vi "CreateClass.vi"(0 "ClassWriterGOOP400.lvclass":refnum<class "ClassWriterGOOP400.lvclass">, 1 "ProjectTreePosition(String or Project Item Ref)":variant, 2 "CreateClassData":T1, 5 "error in (no error)":errorcluster, 6 "KeepLvClassRefOpen(False)":bool, 7 "HeaderToApply (take from VIRef or /use 2D-8bit header, Ignored if not wired)":variant) -> (14 "ClassWriterGOOP400.lvclass":refnum<class "ClassWriterGOOP400.lvclass">, 15 "LVClassLibraryRefnum":refnum<vi>, 16 "TemplateVersionUsed":string, 19 "error out":errorcluster)   [LabVIEW 2012, in "ClassWriterGOOP400.lvclass"]
uses:
  <resource>/Framework/Providers/Open_GDS/ClassProviders/Provider_EndevoGOOP400/ClassWriterGOOP400_class/ClassWriterGOOP400.lvclass
  <resource>/Framework/Providers/Open_GDS/ClassProviders/Provider_BaseClassInterface/CreateClassData.ctl
  <resource>/Framework/Providers/Open_GDS/ClassProviders/Provider_EndevoGOOP400/EndevoG4ProviderName.ctl
  <resource>/Framework/Providers/Open_GDS/ClassProviders/Common/LvClass_class/GDSLvCLass_ClassSettingsType.ctl
  <resource>/Framework/Providers/Open_GDS/ClassProviders/Common/LvClass_class/GDSLvClass_PlugIn.ctl
  <resource>/Framework/Providers/Open_GDS/ClassProviders/Common/LvClass_class/GDSLvClass_PlugInTypes.ctl
  <resource>/Framework/Providers/Open_GDS/ClassProviders/Provider_BaseClassInterface/ClassWriter_class/ClassWriter.lvclass
  <resource>/Framework/Providers/Open_GDS/ClassProviders/Provider_LvNativeClass/ClassWriterNative_class/ClassWriterNative.lvclass
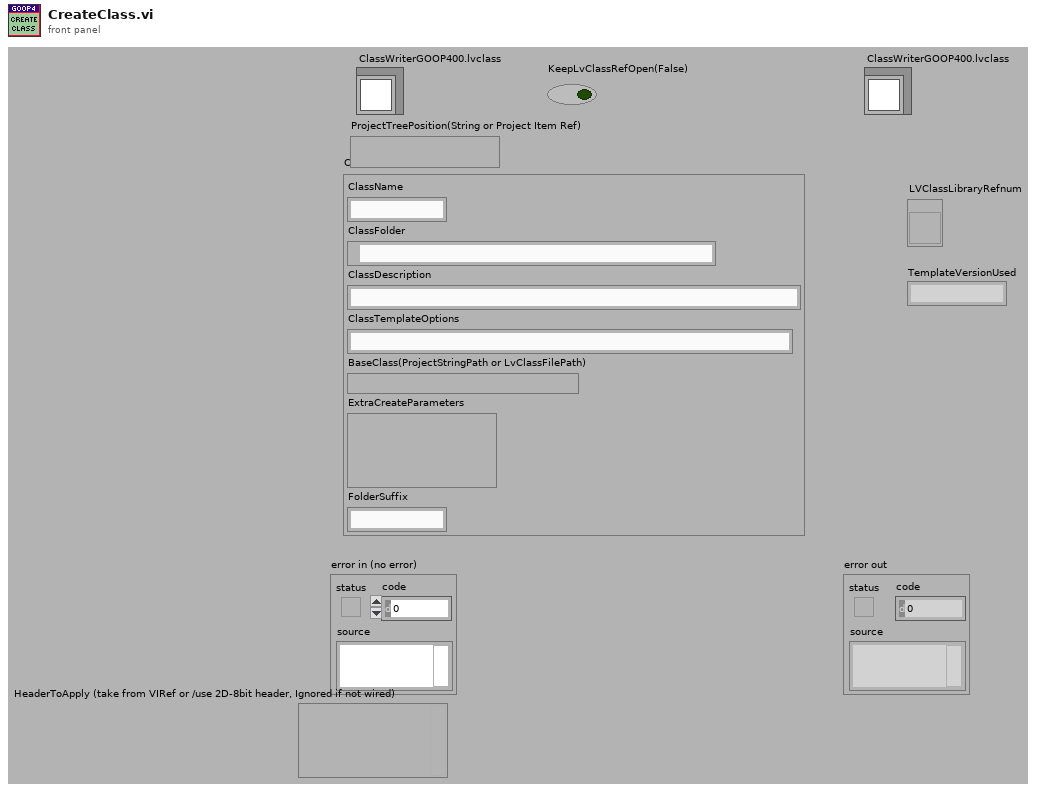
[diagram p1: front panel]
types:
  T1 = typedef "ClassWriter.lvclass/CreateClassData.ctl" = cluster{"ClassName":string, "ClassFolder":path, "ClassDescription":string, "ClassTemplateOptions":string, "BaseClass(ProjectStringPath or LvClassFilePath)":variant, "ExtraCreateParameters":variant, "FolderSuffix":string}
  T2 = cluster{"SubClass":bool, "ClassTemplateFiles":path[], "ClassName":string, "ClassFolder":path, "VIs":refnum<vi>[], "TemplateFolder":path, "ViSubDirs":string[], "TemplateName":string, "BaseClassFolder":path, "RootBaseClassFolder":path, "LvClassPath":path, "ClassRefnum":refnum<vi>, "ProjectRefnum":refnum<vi>, "LvClassFolderPath":path, "BaseClassName":string, "ClassItems":refnum<vi>[], "ViLocked":bool[], "ProjectItemOwner":refnum<vi>, "DeleteFiles":path[], "VIsBefore":refnum<vi>[], "BaseClassPath":path, "BaseConstructorBase":path, "TemplBaseConstructorBase":path, "TemplatePath":path, "TemplateVersion":string, "TemplateParentClass":refnum<vi>, "App":refnum<vi>, "Parent Class":refnum<vi>, "ParentVIs":refnum<vi>[], "TempClass":refnum<vi>}
  T3 = typedef "EndevoG4ProviderName.ctl" = enum16{"EndevoGOOP400"}
  T4 = typedef "GDSLvCLass_ClassSettingsType.ctl" = cluster{"ClassProviderName":string, "ClassTemplateUsed":string, "ClassTemplateVersion":string, "ClassDescription":string, "PlugIns":T5[], "ConnectorPanePattern":string}
  T5 = typedef "GDSLvClass_PlugIn.ctl" = cluster{"Type":T6, "ID":string, "Version":string, "Path":path, "Name":string, "Data":variant}
  T6 = typedef "GDSLvClass_PlugInTypes.ctl" = enum16{"DesignPattern", "MethodTypes"}
  T7 = enum32{"invalid scope", "public", "private", "protected"}
  T8 = enum32{"invalid lock state", "Not Locked", "Locked (No Password)", "Password-protected"}
  T9 = typedef "ClassWriter.lvclass/TemplateSettings.ctl" = cluster{"CommonClassTemplate":bool, "DynamicDispatch":enum8{"False", "True", "Mixed"}, "MustOverride":enum8{"False", "True", "Mixed"}, "MustCallParent":enum8{"False", "True", "Mixed"}, "OnlyNormalMethod":bool, "OnlyPublic":bool}
  T10 = cluster{"Major":u16, "Minor":u16, "Fix":u16, "Build":u16}
  T11 = typedef "Scripting_ConnectorPanePatternType.ctl" = u16
  T12 = typedef "GOOP400_Options.ctl" = cluster{"FlatFolderStructure":bool}
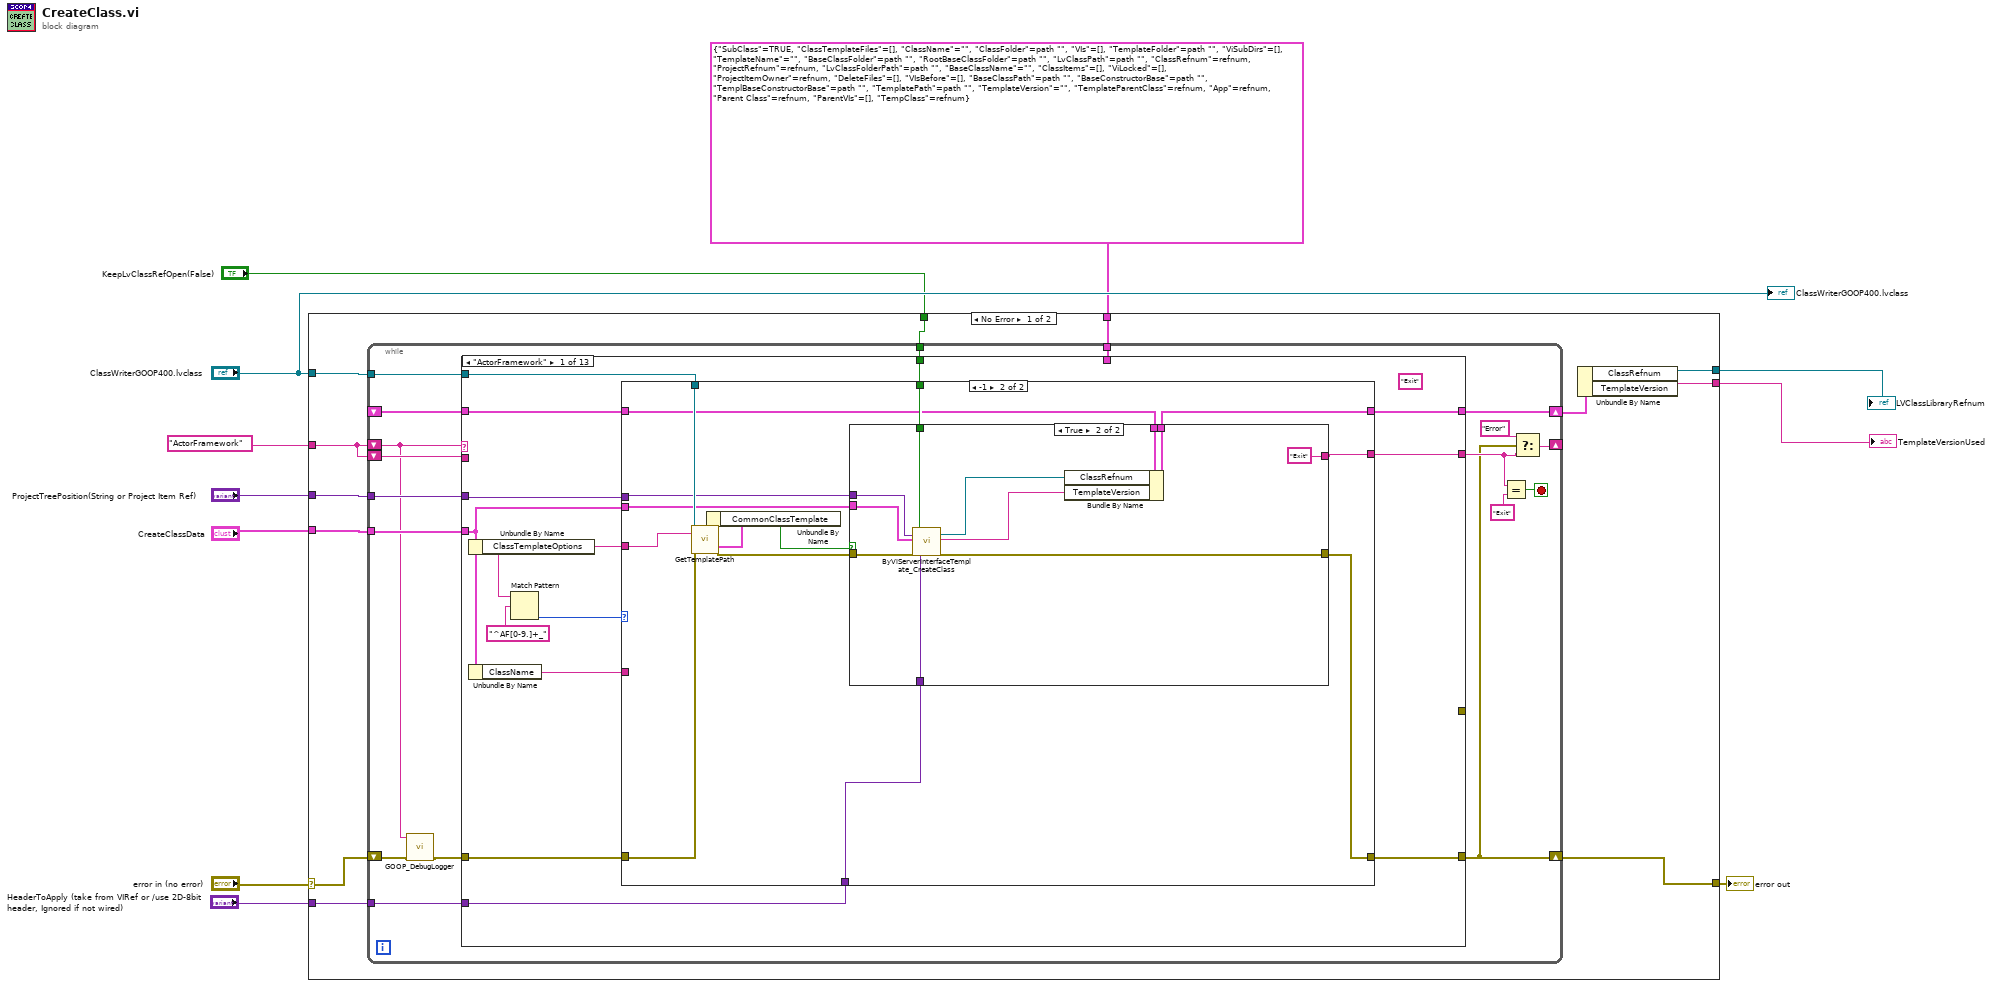
[diagram p0: block diagram]
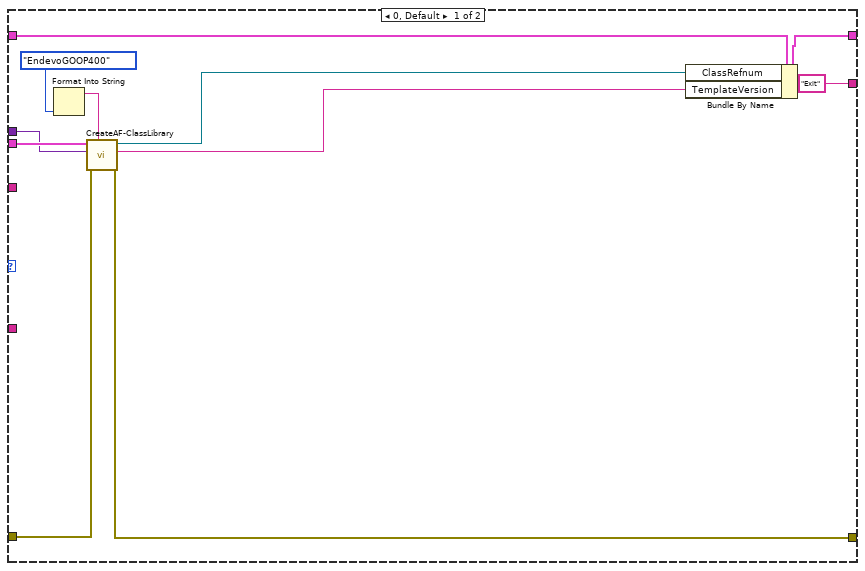
[diagram p2: hidden frame]
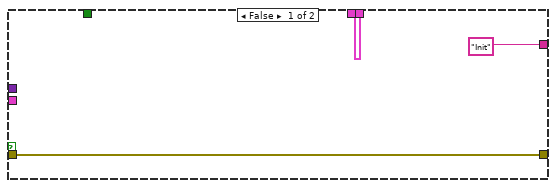
[diagram p3: hidden frame]
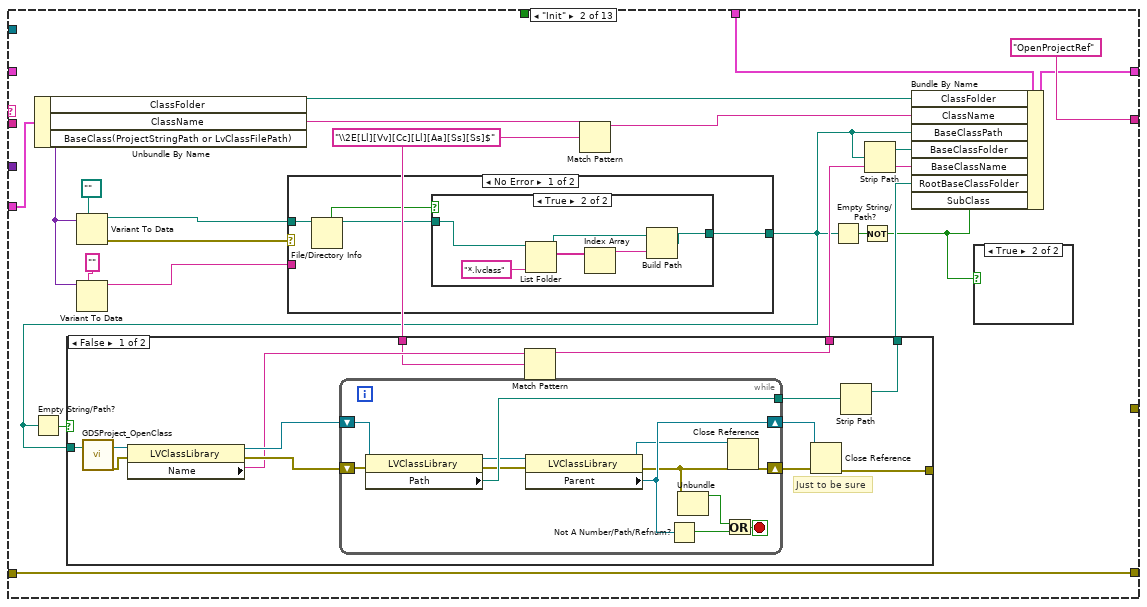
[diagram p4: hidden frame]
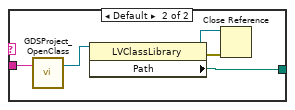
[diagram p9: hidden frame]
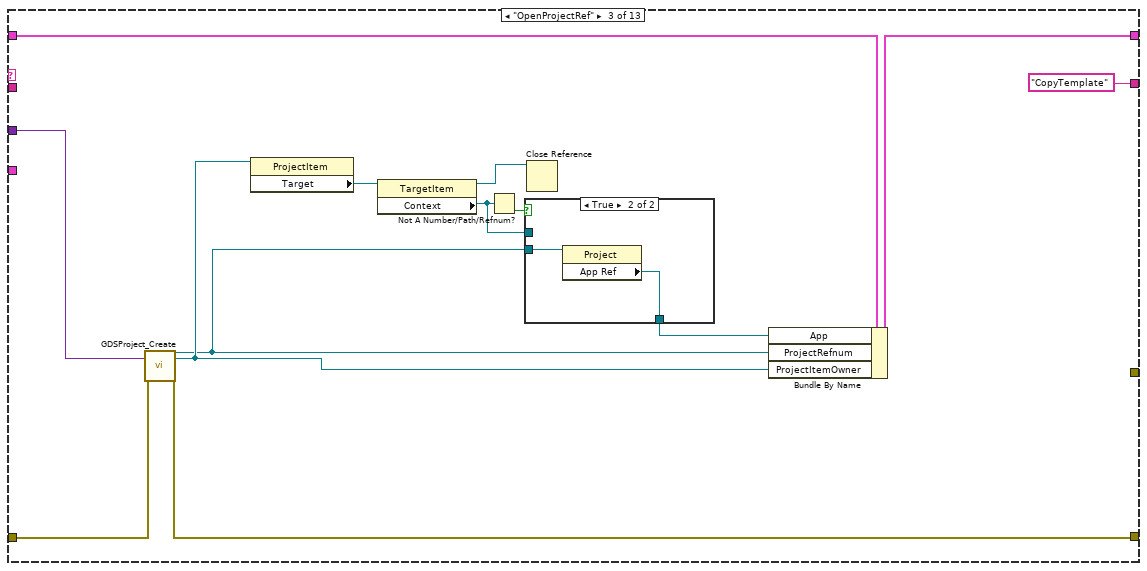
[diagram p10: hidden frame]
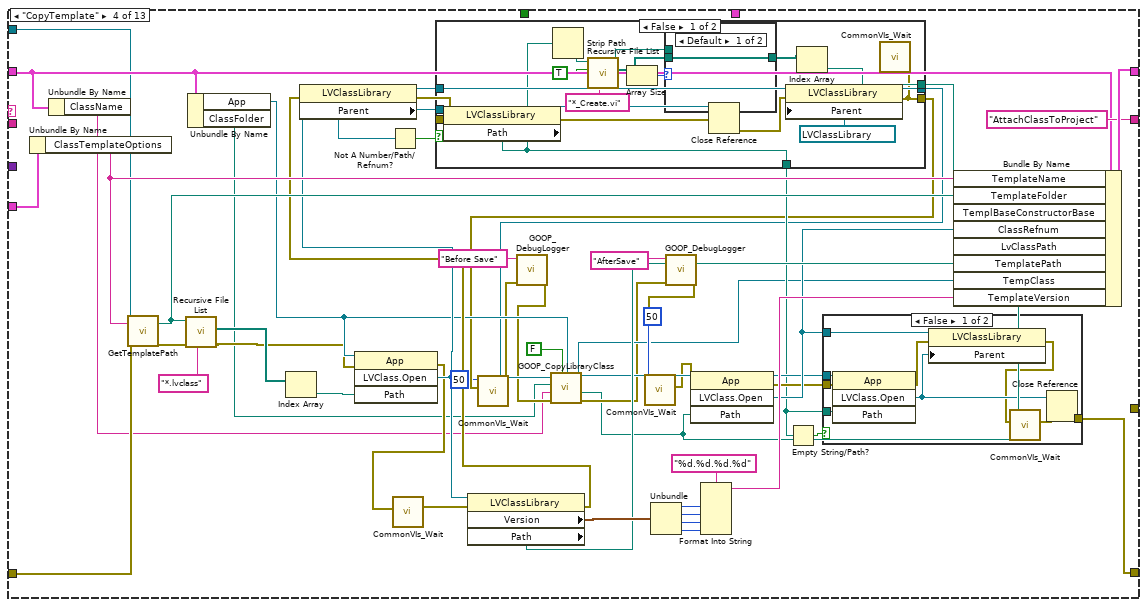
[diagram p12: hidden frame]
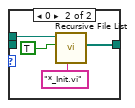
[diagram p14: hidden frame]
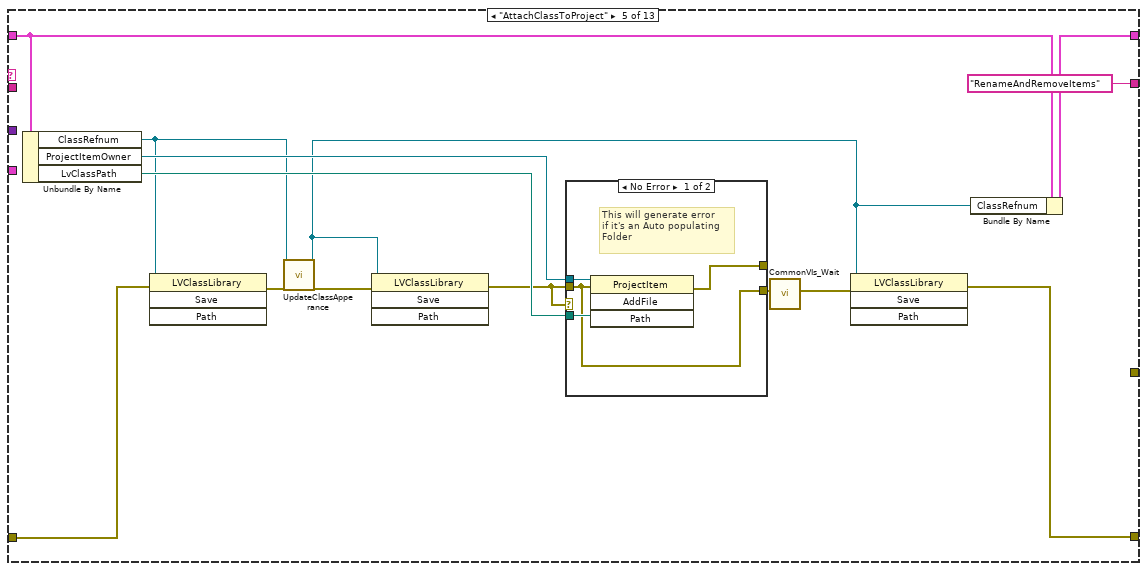
[diagram p16: hidden frame]
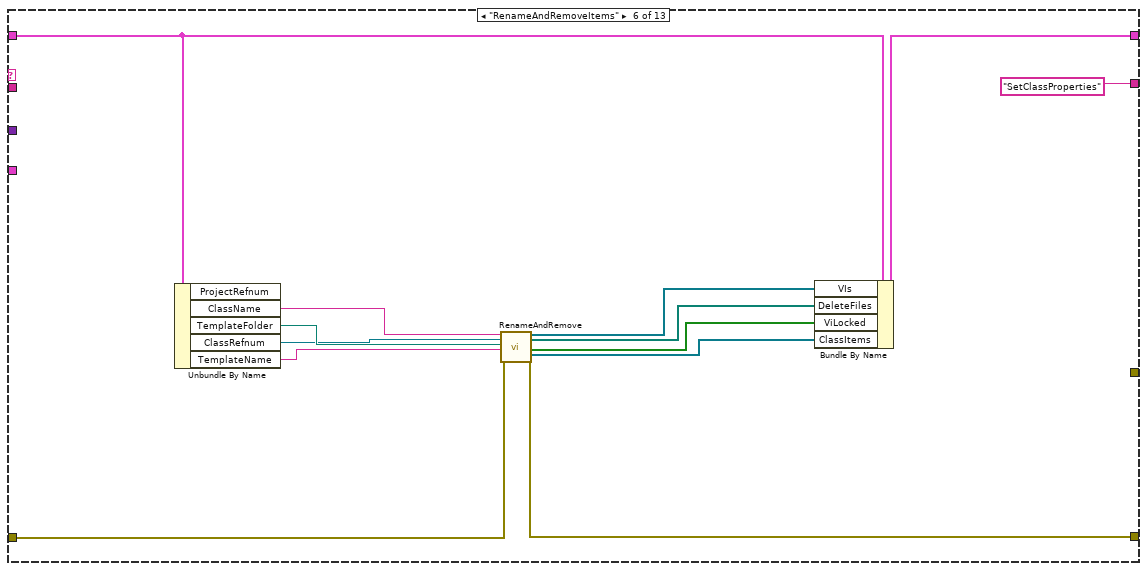
[diagram p18: hidden frame]
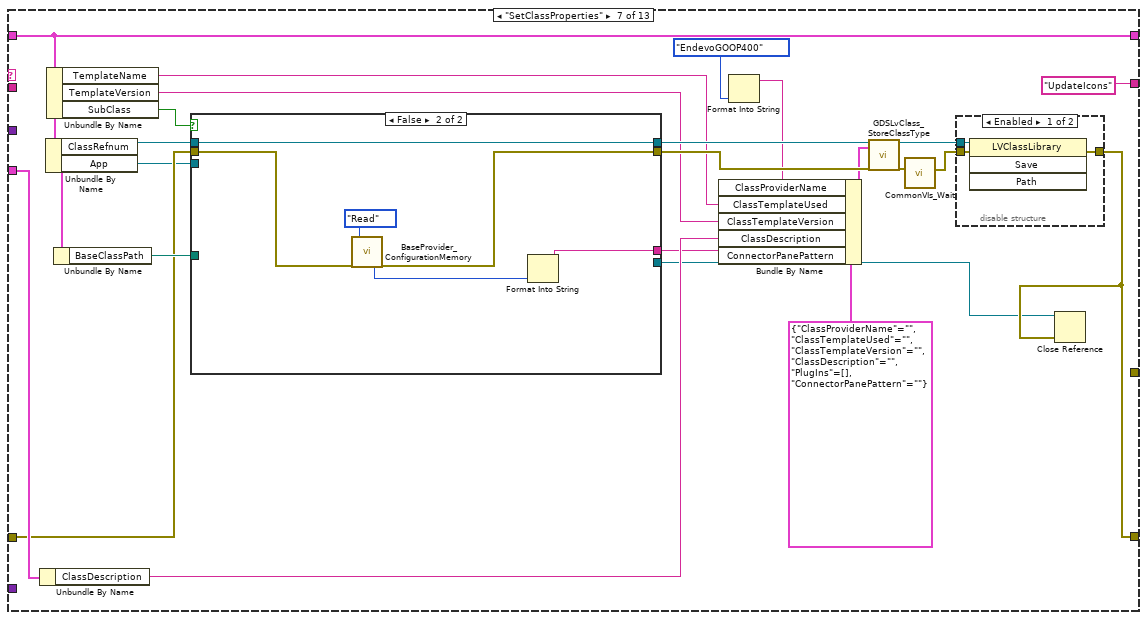
[diagram p19: hidden frame]
diagram:
  n1 = case shown="No Error" "error in (no error)" {
    selector: "error in (no error)" -> [w13 w644]
    tunnel: [w23 w644] -> w11
    tunnel: "ProjectTreePosition(String or Project Item Ref)" -> [w22 _]
    tunnel: "CreateClassData" -> [w21 _]
    tunnel: "ClassWriterGOOP400.lvclass" -> [w20 _]
    tunnel: "HeaderToApply (take from VIRef or /use 2D-8bit header, Ignored if not wired)" -> [w19 _]
    tunnel: "KeepLvClassRefOpen(False)" -> [w18 _]
    tunnel: [w17 _] -> w4
    tunnel: [w16 _] -> w3
    tunnel: T2 {"SubClass"=TRUE, "ClassTemplateFiles"=[], "ClassName"="", "ClassFolder"=path "", "VIs"=[], "TemplateFolder"=path "", "ViSubDirs"=[], "TemplateName"="", "BaseClassFolder"=path "", "RootBaseClassFolder"=path "", "LvClassPath"=path "", "ClassRefnum"=refnum, "ProjectRefnum"=refnum, "LvClassFolderPath"=path "", "BaseClassName"="", "ClassItems"=[], "ViLocked"=[], "ProjectItemOwner"=refnum, "DeleteFiles"=[], "VIsBefore"=[], "BaseClassPath"=path "", "BaseConstructorBase"=path "", "TemplBaseConstructorBase"=path "", "TemplatePath"=path "", "TemplateVersion"="", "TemplateParentClass"=refnum, "App"=refnum, "Parent Class"=refnum, "ParentVIs"=[], "TempClass"=refnum} ("output cluster") -> [w15 _]
    tunnel: "ActorFramework" -> [w12 _]
    frame No Error {
      n2 = while {
        shift-right: [w33] -> w23
        shift-left: w13 -> [w26]
        shift-right: [w37] -> _
        shift-left: w12 -> [w24]
        shift-right: [w40] -> w14
        shift-left: _ -> [w41]
        tunnel: w15 -> [w35]
        tunnel: w22 -> [w32]
        tunnel: w21 -> [w31]
        tunnel: w20 -> [w30]
        shift-left: w12 -> [w29]
        tunnel: w19 -> [w28]
        tunnel: w18 -> [w27]
        stop <- w38 stop-if-true
        n3 = call <resource>:"GOOP_DebugLogger.vi"("error in (no error)"=w26, "State"=w24) -> ("error out"=w25:errorcluster)  [unwired: 9 in]
        n4 = case shown="\"ActorFramework\"" w24 {
          selector: w24 -> [_ _ _ _ _ _ _ _ _ _ _ _ w599]
          tunnel: w41 -> [w55 _ w170 w222 w275 w290 w305 w356 w378 w387 w499 w560 w583]
          tunnel: [w54 w113 w169 w227 w274 w292 w305 w356 w379 w387 w499 w560 w583] -> w40
          tunnel: w25 -> [w50 w116 w168 w218 w269 w287 w306 w349 w375 w401 w520 w562 w600]
          tunnel: [w49 w116 w166 w193 w265 w288 w296 w346 w361 w385 w500 w564 w596] -> w33
          tunnel: [w53 "OpenProjectRef" "CopyTemplate" "AttachClassToProject" "RenameAndRemoveItems" "SetClassProperties" "UpdateIcons" w358 "UpdateVIs" ("t") "AddFolders" "AddFolders" "CloseRefs" "Exit"] -> w34
          tunnel: w35 -> [_ w109 _ _ _ _ _ _ _ _ _ _ _]
          tunnel: w32 -> [w48 _ w167 _ _ _ _ _ _ _ _ _ _]
          tunnel: w31 -> [w46 w108 _ w221 _ _ w313 _ _ _ _ _ _]
          tunnel: w30 -> [w44 _ _ w219 _ _ _ w343 _ _ _ _ _]
          tunnel: w29 -> [_ _ _ _ _ _ _ _ _ _ _ _ w595]
          tunnel: w28 -> [w42 _ _ _ _ _ _ w354 _ _ _ _ _]
          tunnel: w27 -> [w43 _ _ _ _ _ _ _ _ _ _ _ w591]
          tunnel: [_ _ _ _ _ _ _ _ _ _ _ _ w589] -> _
          frame "ActorFramework" {
            (unwired) "Exit"
            n5 = Unbundle By Name(w46) -> ("ClassTemplateOptions"=w47:string)
            n6 = Unbundle By Name(w46) -> ("ClassName"=w45:string)
            n7 = Match Pattern(string=w47, regular expression="^AF[0-9.]+_") -> (offset past match=w51:i32)  [unwired: 1 in, 3 out]
            n8 = case shown="-1" w51 {
              tunnel: w55 -> [w66 w73]
              tunnel: [w65 w72] -> w54
              tunnel: ["Exit" w80] -> w53
              tunnel: w46 -> [w63 w70]
              tunnel: w50 -> [w62 w79]
              tunnel: [w61 w75] -> w49
              tunnel: w48 -> [w58 w71]
              tunnel: w47 -> [_ w77]
              tunnel: w45 -> [_ _]
              tunnel: w44 -> [_ w78]
              tunnel: w43 -> [_ w74]
              tunnel: w42 -> [_ w69]
              frame 0, Default {
                n9 = Format Into String(EndevoG4ProviderName."EndevoGOOP400" ("ProviderName")) -> (resulting string=w60:string)  [unwired: 3 in, 1 out]
                n10 = call <resource>:"CreateAF-ClassLibrary.vi"("Providername"=w60, "error in (no error)"=w62, "ProjectTreePosition(String or Project Item Ref)"=w58, "CreateClassData"=w63) -> ("error out"=w61:errorcluster, "TemplateVersionUsed"=w59:string, "LVClassLibraryRefnum"=w56:refnum<vi>)  [unwired: 5 in]
                n11 = Bundle By Name(cluster=w66, "ClassRefnum"=w56, "TemplateVersion"=w59) -> (w65:T2)
              }
              frame -1 {
                n12 = call-dynamic "GetTemplatePath.vi"("reference in"=w78, "ClassTemplateSubDirectory"=w77, "error in (no error)"=w79) -> ("TemplateSettings"=w68:T9, "error out"=w76:errorcluster)  [unwired: 12 in, 3 out]
                n13 = Unbundle By Name(w68) -> ("CommonClassTemplate"=w67:bool)
                n14 = case shown="True" w67 {
                  tunnel: ["Init" "Exit"] -> w80
                  tunnel: w76 -> [w82 w91]
                  tunnel: [w82 w90] -> w75
                  tunnel: w74 -> [_ w89]
                  tunnel: w73 -> [w81 w88]
                  tunnel: [w81 w87] -> w72
                  tunnel: w71 -> [_ w86]
                  tunnel: w70 -> [_ w85]
                  tunnel: w69 -> [_ w84]
                  frame False {
                  }
                  frame True {
                    n15 = call <resource>:"ByViServerInterfaceTemplate_CreateClass.vi"("ProjectTreePosition(String or Project Item Ref)"=w86, "CreateClassData"=w85, "error in (no error)"=w91, "KeepLvClassRefOpen(False)"=w89, "HeaderToApply (take from VIRef or /use 2D-8bit header, Ignored if not wired)"=w84) -> ("LVClassLibraryRefnum"=w93:refnum<vi>, "TemplateVersionUsed"=w92:string, "error out"=w90:errorcluster)  [unwired: 12 in]
                    n16 = Bundle By Name(cluster=w88, "ClassRefnum"=w93, "TemplateVersion"=w92) -> (w87:T2)
                  }
                }
              }
            }
          }
          frame "Init" {
            w105 = "\\2E[Ll][Vv][Cc][Ll][Aa][Ss][Ss]$" ("regular expression")
            n17 = Unbundle By Name(w108) -> ("ClassFolder"=w102:path, "ClassName"=w101:string, "BaseClass(ProjectStringPath or LvClassFilePath)"=w107:variant)
            n18 = Variant To Data(type=path "" ("path"), Variant=w107) -> (data=w98:path, error out=w99:errorcluster)  [unwired: 1 in]
            n19 = Variant To Data(type="" ("regular expression"), Variant=w107) -> (data=w110:string)  [unwired: 1 in, 1 out]
            n20 = case shown="No Error" w99 {
              tunnel: [w144 w152] -> w96
              tunnel: w110 -> [_ w153]
              tunnel: w98 -> [w143 _]
              frame No Error {
                n21 = File/Directory Info(path=w143) -> (path out=w141:path, directory=w142:bool)  [unwired: 1 in, 5 out]
                n22 = case shown="True" w142 {
                  tunnel: [w145 w147] -> w144
                  tunnel: w141 -> [w145 w146]
                  frame False {
                  }
                  frame True {
                    n23 = List Folder(path=w146, pattern="*.lvclass") -> (path out=w148:path, filenames=w150:string[])  [unwired: 2 in, 2 out]
                    n24 = Index Array(array=w150) -> (element=w149:string)  [unwired: 1 in]
                    n25 = Build Path(base path=w148, name or relative path=w149) -> (appended path=w147:path)
                  }
                }
              }
              frame Error {
                n26 = case shown="\"\"" w153 {
                  tunnel: w153 -> [_ w158]
                  tunnel: [_ w154] -> w152
                  frame "" {
                  }
                  frame Default {
                    n27 = call <resource>:"GDSProject_OpenClass.vi"("ClassPath(FilePath/ProjectTreePath/LvCLassRef)"=w158) -> ("LVClass.Open"=w157:refnum<vi>)  [unwired: 16 in, 2 out]
                    n28 = property class="LVClassLibrary"(reference=w157) -> (reference out=w155:refnum<vi>, error out=w156:errorcluster, "Path"=w154:path)  [unwired: 1 in]
                    n29 = Close Reference(reference=w155, error in (no error)=w156) -> ()  [unwired: 1 out]
                  }
                }
              }
            }
            n30 = Empty String/Path?(string/path=w96) -> (empty?=w103:bool)
            n31 = case shown="False" w103 {
              tunnel: [w126 _] -> w106
              tunnel: w105 -> [w120 _]
              tunnel: [w119 _] -> w104
              tunnel: w96 -> [w118 _]
              tunnel: [w117 _] -> _
              frame False {
                # "Just to be sure"
                n32 = call <resource>:"GDSProject_OpenClass.vi"("ClassPath(FilePath/ProjectTreePath/LvCLassRef)"=w118) -> ("LVClass.Open"=w123:refnum<vi>, "error out"=w125:errorcluster)  [unwired: 16 in, 1 out]
                n33 = property class="LVClassLibrary"(reference=w123, error in=w125) -> (reference out=w122:refnum<vi>, error out=w124:errorcluster, "Name"=w121:string)
                n34 = while {
                  shift-right: [w137] -> w129
                  shift-left: w124 -> [w132]
                  shift-right: [w138] -> w128
                  shift-left: w122 -> [w140]
                  tunnel: [w139] -> w127
                  stop <- w134 stop-if-true
                  n35 = property class="LVClassLibrary"(reference=w140, error in=w132) -> (reference out=w130:refnum<vi>, error out=w131:errorcluster, "Path"=w139:path)
                  n36 = property class="LVClassLibrary"(reference=w130, error in=w131) -> (reference out=w133:refnum<vi>, error out=w137:errorcluster, "Parent"=w138:refnum<vi>)
                  n37 = Not A Number/Path/Refnum?(number/path/refnum=w138) -> (NaN/Path/Refnum?=w135:bool)
                  n38 = Unbundle(w137) -> ("status"=w136:bool)  [unwired: 2 out]
                  n39 = Or(x=w136, y=w135) -> (x .or. y?=w134:bool)
                  n40 = Close Reference(reference=w133) -> ()  [unwired: 1 in, 1 out]
                }
                n41 = Match Pattern(string=w121, regular expression=w120) -> (before substring=w119:string)  [unwired: 1 in, 3 out]
                n42 = Close Reference(reference=w128, error in (no error)=w129) -> (error out=w117:errorcluster)
                n43 = Strip Path(path=w127) -> (stripped path=w126:path)  [unwired: 1 out]
              }
              frame True {
              }
            }
            n44 = Match Pattern(string=w101, regular expression=w105) -> (before substring=w114:string)  [unwired: 1 in, 3 out]
            n45 = Empty String/Path?(string/path=w96) -> (empty?=w97:bool)
            n46 = Not(x=w97) -> (.not. x?=w95:bool)
            n47 = Strip Path(path=w96) -> (stripped path=w100:path)  [unwired: 1 out]
            n48 = Bundle By Name(cluster=w109, "ClassFolder"=w102, "ClassName"=w114, "BaseClassPath"=w96, "BaseClassFolder"=w100, "BaseClassName"=w104, "RootBaseClassFolder"=w106, "SubClass"=w95) -> (w113:T2)
            n49 = case shown="True" w95 {
              frame False {
              }
              frame True {
              }
            }
          }
          frame "OpenProjectRef" {
            n50 = call <resource>:"GDSProject_Create.vi"("ProjectTreePosition(String or Project Item Ref)"=w167, "error in (no error)"=w168) -> ("Project Refnum"=w160:refnum<vi>, "Project Item"=w161:refnum<vi>, "error out"=w166:errorcluster)  [unwired: 15 in]
            n51 = property class="ProjectItem"(reference=w161) -> ("Target"=w165:refnum<vi>)  [unwired: 1 in, 2 out]
            n52 = property class="TargetItem"(reference=w165) -> (reference out=w164:refnum<vi>, "Context"=w162:refnum<vi>)  [unwired: 1 in, 1 out]
            n53 = Not A Number/Path/Refnum?(number/path/refnum=w162) -> (NaN/Path/Refnum?=w163:bool)
            n54 = case shown="True" w163 {
              tunnel: [w172 w174] -> w159
              tunnel: w160 -> [_ w173]
              tunnel: w162 -> [w172 _]
              frame False {
              }
              frame True {
                n55 = property class="Project"(reference=w173) -> ("App Ref"=w174:refnum<vi>)  [unwired: 1 in, 2 out]
              }
            }
            n56 = Close Reference(reference=w164) -> ()  [unwired: 1 in, 1 out]
            n57 = Bundle By Name(cluster=w170, "App"=w159, "ProjectRefnum"=w160, "ProjectItemOwner"=w161) -> (w169:T2)
          }
          frame "CopyTemplate" {
            n58 = Unbundle By Name(w221) -> ("ClassTemplateOptions"=w220:string)
            n59 = Unbundle By Name(w222) -> ("ClassName"=w177:string)
            n60 = call-dynamic "GetTemplatePath.vi"("reference in"=w219, "ClassTemplateSubDirectory"=w220, "error in (no error)"=w218) -> ("FolderPathOut"=w216:path, "error out"=w217:errorcluster)  [unwired: 12 in, 3 out]
            n61 = call <vilib>:"Recursive File List.vi"("pattern"="*.lvclass", "error in (no error)"=w217, "Folder Path"=w216) -> ("error out"=w194:errorcluster, "All Files in Dir"=w224:path[])  [unwired: 4 in, 3 out]
            n62 = Unbundle By Name(w222) -> ("App"=w195:refnum<vi>, "ClassFolder"=w176:path)
            n63 = Index Array(array=w224) -> (element=w223:path)  [unwired: 1 in]
            n64 = invoke class="App" method="LVClass.Open"(reference=w195, error in=w194, "Path"=w223) -> (error out=w190:errorcluster, "LVClass.Open"=w202:refnum<vi>)  [unwired: 1 in, 2 out]
            n65 = call <resource>:"CommonVIs_Wait.vi"("error in"=w190) -> ("error out"=w191:errorcluster)  [unwired: 9 in]
            n66 = property class="LVClassLibrary"(reference=w202, error in=w191) -> (error out=w203:errorcluster, "Version"=w215:T10, "Path"=w209:path)  [unwired: 1 out]
            n67 = property class="LVClassLibrary"(reference=w202, error in=w203) -> (reference out=w207:refnum<vi>, error out=w199:errorcluster, "Parent"=w200:refnum<vi>)
            n68 = Not A Number/Path/Refnum?(number/path/refnum=w200) -> (NaN/Path/Refnum?=w198:bool)
            n69 = case shown="False" w198 {
              tunnel: w207 -> [w252 w261]
              tunnel: [w251 w261] -> w181
              tunnel: [w238 w262] -> w189
              tunnel: [w248 _] -> w201
              tunnel: w200 -> [w246 _]
              tunnel: w199 -> [w245 w262]
              tunnel: [w243 _] -> w197
              frame False {
                n70 = property class="LVClassLibrary"(reference=w246, error in=w245) -> (reference out=w254:refnum<vi>, error out=w255:errorcluster, "Path"=w243:path)
                n71 = Strip Path(path=w243) -> (stripped path=w247:path)  [unwired: 1 out]
                n72 = call <vilib>:"Recursive File List.vi"("pattern"="*_Create.vi", "Treat LLBs as Folders?"=TRUE, "Folder Path"=w247) -> ("All Files in Dir"=w239:path[], "dup Folder Path"=w240:path)  [unwired: 4 in, 3 out]
                n73 = Array Size(array=w239) -> (size(s)=w242:i32)
                n74 = case shown="Default" w242 {
                  tunnel: w239 -> [w256 _]
                  tunnel: [w256 w257] -> w241
                  tunnel: w240 -> [_ w258]
                  frame Default {
                  }
                  frame 0 {
                    n75 = call <vilib>:"Recursive File List.vi"("pattern"="*_Init.vi", "Treat LLBs as Folders?"=TRUE, "Folder Path"=w258) -> ("All Files in Dir"=w257:path[])  [unwired: 4 in, 4 out]
                  }
                }
                n76 = Close Reference(reference=w254, error in (no error)=w255) -> (error out=w253:errorcluster)
                n77 = property class="LVClassLibrary"(reference=w252, error in=w253, "Parent"=refnum<vi> refnum ("Parent Class")) -> (reference out=w251:refnum<vi>, error out=w238:errorcluster)
                n78 = Index Array(array=w241) -> (element=w248:path)  [unwired: 1 in]
                n79 = call <resource>:"CommonVIs_Wait.vi"("error in"=w238) -> ()  [unwired: 9 in, 1 out]
              }
              frame True {
              }
            }
            n80 = call <resource>:"CommonVIs_Wait.vi"("error in"=w189, "Wait(150ms)"=u32 50) -> ("error out"=w186:errorcluster)  [unwired: 8 in]
            n81 = call <resource>:"GOOP_DebugLogger.vi"("error in (no error)"=w186, "State"="Before Save") -> ("error out"=w180:errorcluster)  [unwired: 9 in]
            n82 = call <resource>:"GOOP_CopyLibraryClass.vi"("ManualCopy"=FALSE, "error in"=w180, "New Name"=w177, "Path"=w176, "LVClassIn"=w181) -> ("error out"=w179:errorcluster, "New Lib Path"=w178:path, "LVClassOut"=w182:refnum<vi>)  [unwired: 4 in]
            n83 = Unbundle(w215) -> ("Major"=w213:u16, "Minor"=w212:u16, "Fix"=w211:u16, "Build"=w210:u16)
            n84 = call <resource>:"GOOP_DebugLogger.vi"("error in (no error)"=w179, "State"="AfterSave") -> ("error out"=w184:errorcluster)  [unwired: 9 in]
            n85 = call <resource>:"CommonVIs_Wait.vi"("error in"=w184, "Wait(150ms)"=u32 50) -> ("error out"=w192:errorcluster)  [unwired: 8 in]
            n86 = invoke class="App" method="LVClass.Open"(reference=w195, error in=w192, "Path"=w178) -> (reference out=w205:refnum<vi>, error out=w204:errorcluster, "LVClass.Open"=w206:refnum<vi>)  [unwired: 1 in, 1 out]
            n87 = Format Into String(format string="%d.%d.%d.%d", w213, w212, w211, w210) -> (resulting string=w208:string)  [unwired: 2 in, 1 out]
            n88 = Empty String/Path?(string/path=w197) -> (empty?=w196:bool)
            n89 = case shown="False" w196 {
              tunnel: w206 -> [w236 _]
              tunnel: w205 -> [w235 _]
              tunnel: w204 -> [w234 w237]
              tunnel: [w233 w237] -> w193
              tunnel: w197 -> [w231 _]
              frame False {
                n90 = invoke class="App" method="LVClass.Open"(reference=w235, error in=w234, "Path"=w231) -> (error out=w230:errorcluster, "LVClass.Open"=w232:refnum<vi>)  [unwired: 1 in, 2 out]
                n91 = property class="LVClassLibrary"(reference=w236, error in=w230, "Parent"=w232) -> (error out=w228:errorcluster)  [unwired: 1 out]
                n92 = call <resource>:"CommonVIs_Wait.vi"("error in"=w228) -> ("error out"=w229:errorcluster)  [unwired: 9 in]
                n93 = Close Reference(reference=w232, error in (no error)=w229) -> (error out=w233:errorcluster)
              }
              frame True {
              }
            }
            n94 = Bundle By Name(cluster=w222, "TemplateName"=w220, "TemplateFolder"=w216, "TemplBaseConstructorBase"=w201, "ClassRefnum"=w206, "LvClassPath"=w178, "TemplatePath"=w209, "TempClass"=w182, "TemplateVersion"=w208) -> (w227:T2)
          }
          frame "AttachClassToProject" {
            n95 = Unbundle By Name(w275) -> ("ClassRefnum"=w268:refnum<vi>, "ProjectItemOwner"=w276:refnum<vi>, "LvClassPath"=w272:path)
            n96 = invoke class="LVClassLibrary" method="Save"(reference=w268, error in=w269) -> (error out=w270:errorcluster)  [unwired: 2 in, 3 out]
            n97 = call <resource>:"UpdateClassApperance.vi"("ClassRefIn"=w268, "error in (no error)"=w270) -> ("ClassRefOut"=w263:refnum<vi>, "error out"=w267:errorcluster)  [unwired: 16 in]
            n98 = invoke class="LVClassLibrary" method="Save"(reference=w263, error in=w267) -> (error out=w264:errorcluster)  [unwired: 2 in, 3 out]
            n99 = case shown="No Error" w264 {
              tunnel: w276 -> [w280 _]
              tunnel: w272 -> [w279 _]
              tunnel: [w278 w281] -> w271
              tunnel: w264 -> [w278 w281]
              tunnel: [w277 _] -> _
              frame No Error {
                # "This will generate error\nif it's an Auto populating\nFolder"
                n100 = invoke class="ProjectItem" method="AddFile"(reference=w280, error in=w278, "Path"=w279) -> (error out=w277:errorcluster)  [unwired: 1 in, 3 out]
              }
              frame Error {
              }
            }
            n101 = call <resource>:"CommonVIs_Wait.vi"("error in"=w271) -> ("error out"=w266:errorcluster)  [unwired: 9 in]
            n102 = invoke class="LVClassLibrary" method="Save"(reference=w263, error in=w266) -> (error out=w265:errorcluster)  [unwired: 2 in, 3 out]
            n103 = Bundle By Name(cluster=w275, "ClassRefnum"=w263) -> (w274:T2)
          }
          frame "RenameAndRemoveItems" {
            n104 = Unbundle By Name(w290) -> ("ClassName"=w294:string, "TemplateFolder"=w291:path, "ClassRefnum"=w289:refnum<vi>, "TemplateName"=w282:string)  [unwired: 1 out]
            n105 = call <resource>:"RenameAndRemove.vi"("ClassName"=w294, "ClassRefnum"=w289, "TemplateFolder"=w291, "TemplateName"=w282, "error in"=w287) -> ("ViRefsOut"=w293:refnum<vi>[], "DeleteFiles"=w286:path[], "ItemLocked"=w285:bool[], "Items"=w284:refnum<vi>[], "error out"=w288:errorcluster)  [unwired: 10 in]
            n106 = Bundle By Name(cluster=w290, "VIs"=w293, "DeleteFiles"=w286, "ViLocked"=w285, "ClassItems"=w284) -> (w292:T2)
          }
          frame "SetClassProperties" {
            n107 = Unbundle By Name(w313) -> ("ClassDescription"=w309:string)
            n108 = Unbundle By Name(w305) -> ("ClassRefnum"=w307:refnum<vi>, "App"=w301:refnum<vi>)
            n109 = Unbundle By Name(w305) -> ("TemplateName"=w308:string, "TemplateVersion"=w302:string, "SubClass"=w317:bool)
            n110 = Unbundle By Name(w305) -> ("BaseClassPath"=w316:path)
            n111 = case shown="False" w317 {
              tunnel: w307 -> [w325 w342]
              tunnel: [w336 w342] -> w315
              tunnel: w306 -> [w329 w338]
              tunnel: [w335 w337] -> w314
              tunnel: w316 -> [w334 _]
              tunnel: w301 -> [w330 _]
              tunnel: [w331 w339] -> w300
              tunnel: [w323 _] -> w295
              frame True {
                n112 = invoke class="LVClassLibrary" method="Save"(reference=w325) -> (reference out=w324:refnum<vi>)  [unwired: 3 in, 3 out]
                n113 = invoke class="App" method="LVClass.Open"(reference=w330, error in=w329, "Path"=w334) -> (error out=w328:errorcluster, "LVClass.Open"=w333:refnum<vi>)  [unwired: 1 in, 2 out]
                n114 = call <resource>:"CommonVIs_Wait.vi"("error in"=w328) -> ("error out"=w327:errorcluster)  [unwired: 9 in]
                n115 = call <resource>:"GDSLvClass_ReadClassType.vi"("Class Refnum In"=w333, "error in (no error)"=w327) -> ("Class Refnum Out"=w323:refnum<vi>, "ClassSettings"=w332:T4, "error out"=w326:errorcluster)  [unwired: 15 in]
                n116 = Unbundle By Name(w332) -> ("ConnectorPanePattern"=w331:string)
                n117 = invoke class="LVClassLibrary" method="Save"(reference=w323) -> (reference out=w322:refnum<vi>)  [unwired: 3 in, 3 out]
                n118 = property class="LVClassLibrary"(reference=w324, error in=w326, "Parent"=w322) -> (reference out=w336:refnum<vi>, error out=w335:errorcluster)
              }
              frame False {
                n119 = call <resource>:"BaseProvider_ConfigurationMemory.vi"("error in (no error)"=w338, "Action"=enum16{"Read", "Load", "Save"}."Read") -> ("PatternOut"=w341:T11, "error out"=w337:errorcluster)  [unwired: 11 in, 5 out]
                n120 = Format Into String(w341) -> (resulting string=w339:string)  [unwired: 3 in, 1 out]
              }
            }
            n121 = Format Into String(EndevoG4ProviderName."EndevoGOOP400" ("ProviderName")) -> (resulting string=w310:string)  [unwired: 3 in, 1 out]
            n122 = Bundle By Name(cluster=T4 {"ClassProviderName"="", "ClassTemplateUsed"="", "ClassTemplateVersion"="", "ClassDescription"="", "PlugIns"=[], "ConnectorPanePattern"=""} ("ClassSettings"), "ClassProviderName"=w310, "ClassTemplateUsed"=w308, "ClassTemplateVersion"=w302, "ClassDescription"=w309, "ConnectorPanePattern"=w300) -> (w311:T4)
            n123 = call <resource>:"GDSLvClass_StoreClassType.vi"("Class Refnum In"=w315, "ClassSettings"=w311, "error in (no error)"=w314) -> ("Class Refnum Out"=w299:refnum<vi>, "error out"=w298:errorcluster)  [unwired: 15 in]
            n124 = call <resource>:"CommonVIs_Wait.vi"("error in"=w298) -> ("error out"=w297:errorcluster)  [unwired: 9 in]
            n125 = disable-structure shown="Enabled" {
              disable-tunnel: [w320 w321] -> w296
              disable-tunnel: w299 -> [w319 _]
              disable-tunnel: w297 -> [w318 w321]
              frame Enabled {
                n126 = invoke class="LVClassLibrary" method="Save"(reference=w319, error in=w318) -> (error out=w320:errorcluster)  [unwired: 2 in, 3 out]
              }
              frame Disabled {
              }
            }
            n127 = Close Reference(reference=w295, error in (no error)=w296) -> ()  [unwired: 1 out]
          }
          frame "UpdateIcons" {
            n128 = Unbundle By Name(w356) -> ("ClassRefnum"=w355:refnum<vi>)
            n129 = Unbundle By Name(w356) -> ("SubClass"=w360:bool, "ClassName"=w357:string)
            n130 = call-dynamic "ProgressWindow.vi"("ClassWriter in"=w343, "Message(Exit)"="Hide", "error in (no error)"=w349) -> ("ClassWriter out"=w344:refnum<class "ClassWriterGOOP400.lvclass">, "error out"=w348:errorcluster)  [unwired: 15 in]
            n131 = Empty String/Path?(string/path=w354) -> (empty?=w353:bool)
            n132 = Not(x=w353) -> (.not. x?=w352:bool)
            n133 = call <resource>:"GDSLvIcon_DialogUpdateClass.vi"("ClassPath(FilePath/ProjectTreePath/LvCLassRef)"=w355, "ClassName"=w357, "AutoUpdate"=w352, "error in (no error)"=w348, "HeaderToApply (take from VIRef or /use 2D-8bit header, Ignored if not wired)"=w354) -> ("error out"=w347:errorcluster)  [unwired: 14 in]
            n134 = Select(t="GetDerivedClassConstructor", s=w360, f="AddFolders") -> (s? t:f=w358:string)
            n135 = call-dynamic "ProgressWindow.vi"("ClassWriter in"=w344, "Message(Exit)"="UnHide", "error in (no error)"=w347) -> ("error out"=w346:errorcluster)  [unwired: 15 in, 1 out]
          }
          frame "GetDerivedClassConstructor" {
            # "USE BASE CLASS PATH"
            n136 = Unbundle By Name(w378) -> ("ClassRefnum"=w376:refnum<vi>)
            n137 = property class="LVClassLibrary"(reference=w376, error in=w375) -> (error out=w372:errorcluster, "Parent"=w364:refnum<vi>)  [unwired: 1 out]
            n138 = property class="LVClassLibrary"(reference=w364, error in=w372) -> (reference out=w363:refnum<vi>, error out=w362:errorcluster, "Path"=w370:path)
            n139 = Strip Path(path=w370) -> (stripped path=w369:path)  [unwired: 1 out]
            n140 = call <vilib>:"Recursive File List.vi"("pattern"="*_Create.vi", "Treat LLBs as Folders?"=TRUE, "Folder Path"=w369) -> ("All Files in Dir"=w367:path[], "dup Folder Path"=w365:path)  [unwired: 4 in, 3 out]
            n141 = Close Reference(reference=w363, error in (no error)=w362) -> (error out=w361:errorcluster)
            n142 = Array Size(array=w367) -> (size(s)=w368:i32)
            n143 = case shown="0" w368 {
              tunnel: w367 -> [w380 _]
              tunnel: [w380 w381] -> w366
              tunnel: w365 -> [_ w382]
              frame Default {
              }
              frame 0 {
                n144 = call <vilib>:"Recursive File List.vi"("pattern"="*_Init.vi", "Treat LLBs as Folders?"=TRUE, "Folder Path"=w382) -> ("All Files in Dir"=w381:path[])  [unwired: 4 in, 4 out]
              }
            }
            n145 = Index Array(array=w366) -> (element=w371:path)  [unwired: 1 in]
            n146 = Bundle By Name(cluster=w378, "BaseConstructorBase"=w371) -> (w379:T2)
          }
          frame "UpdateVIs" {
            (unwired) "AnyProtectedAttributesToUpdate?"
            # "This is a sub class, replace all BaseClass References with Select base class.\nIf base not equal to root, also replace BaseClass ObjectRef with Root-Base ObjectRef"
            n147 = Unbundle By Name(w387) -> ("TemplBaseConstructorBase"=w399:path, "BaseConstructorBase"=w398:path)
            n148 = Unbundle By Name(w387) -> ("VIs"=w402:refnum<vi>[])
            n149 = call <resource>:"CreateVINamesToReplace.vi"("Foldername"="utils" ("name or relative path"), "NewVIName"="_New.vi" ("string"), "BaseConstructorBase"=w398, "TemplBaseConstructorBase"=w399) -> ("NewVIName"=w395:path, "OldVIName"=w396:path)  [unwired: 5 in]
            n150 = call <resource>:"CreateVINamesToReplace.vi"("NewVIName"="_Init.vi" ("string"), "BaseConstructorBase"=w398, "TemplBaseConstructorBase"=w399) -> ("NewVIName"=w391:path, "OldVIName"=w392:path)  [unwired: 6 in]
            n151 = call <resource>:"CreateVINamesToReplace.vi"("NewVIName"="_CleanUp.vi" ("string"), "BaseConstructorBase"=w398, "TemplBaseConstructorBase"=w399) -> ("NewVIName"=w388:path, "OldVIName"=w389:path)  [unwired: 6 in]
            n152 = for {
              shift-right: [w428] -> w385
              shift-left: w401 -> [w425]
              tunnel: w402 -> [w419] mode=indexing
              tunnel: w399 -> [w427]
              tunnel: w398 -> [w426]
              tunnel: w396 -> [w418]
              tunnel: w395 -> [w417]
              tunnel: w392 -> [w411]
              tunnel: w391 -> [w410]
              tunnel: w389 -> [w406]
              tunnel: w388 -> [w405]
              n153 = property class="VI"(reference=w419) -> ("Name"=w404:string)  [unwired: 1 in, 2 out]
              n154 = Match Pattern(string=w404, regular expression="_Create.vi") -> (offset past match=w424:i32)  [unwired: 1 in, 3 out]
              n155 = Match Pattern(string=w404, regular expression="_New.vi") -> (offset past match=w422:i32)  [unwired: 1 in, 3 out]
              n156 = Match Pattern(string=w404, regular expression="_Init.vi") -> (offset past match=w415:i32)  [unwired: 1 in, 3 out]
              n157 = Match Pattern(string=w404, regular expression="_CleanUp.vi") -> (offset past match=w408:i32)  [unwired: 1 in, 3 out]
              n158 = Greater Or Equal To 0?(x=w424) -> (x >= 0?=w413:bool)
              n159 = Greater Or Equal To 0?(x=w422) -> (x >= 0?=w421:bool)
              n160 = Greater Or Equal To 0?(x=w415) -> (x >= 0?=w412:bool)
              n161 = Greater Or Equal To 0?(x=w408) -> (x >= 0?=w407:bool)
              n162 = Compound Arithmetic op=OR(w413, w421, w412, w407) -> (w420:bool)
              n163 = case shown="True" w420 {
                tunnel: w425 -> [w429 w445]
                tunnel: [w429 w444] -> w428
                tunnel: w419 -> [_ w443]
                tunnel: w427 -> [_ w441]
                tunnel: w426 -> [_ w440]
                tunnel: w421 -> [_ w442]
                tunnel: w418 -> [_ w437]
                tunnel: w417 -> [_ w436]
                tunnel: w412 -> [_ w435]
                tunnel: w411 -> [_ w434]
                tunnel: w410 -> [_ w433]
                tunnel: w407 -> [_ w432]
                tunnel: w406 -> [_ w431]
                tunnel: w405 -> [_ w430]
                frame False {
                }
                frame True {
                  n164 = case shown="False" w442 {
                    tunnel: w441 -> [w454 _]
                    tunnel: w440 -> [w452 _]
                    tunnel: [w453 w470] -> w439
                    tunnel: [w451 w469] -> w438
                    tunnel: w437 -> [_ w470]
                    tunnel: w436 -> [_ w469]
                    tunnel: w435 -> [w455 _]
                    tunnel: w434 -> [w450 _]
                    tunnel: w433 -> [w449 _]
                    tunnel: w432 -> [w448 _]
                    tunnel: w431 -> [w447 _]
                    tunnel: w430 -> [w446 _]
                    frame False {
                      n165 = case shown="False" w455 {
                        tunnel: w454 -> [w461 _]
                        tunnel: [w458 w468] -> w453
                        tunnel: w452 -> [w459 _]
                        tunnel: [w460 w467] -> w451
                        tunnel: w450 -> [_ w468]
                        tunnel: w449 -> [_ w467]
                        tunnel: w448 -> [w462 _]
                        tunnel: w447 -> [w457 _]
                        tunnel: w446 -> [w456 _]
                        frame False {
                          n166 = case shown="True" w462 {
                            tunnel: [w464 w466] -> w458
                            tunnel: w461 -> [w464 _]
                            tunnel: [w463 w465] -> w460
                            tunnel: w459 -> [w463 _]
                            tunnel: w457 -> [_ w466]
                            tunnel: w456 -> [_ w465]
                            frame False {
                            }
                            frame True {
                            }
                          }
                        }
                        frame True {
                        }
                      }
                    }
                    frame True {
                    }
                  }
                  n167 = while {
                    tunnel: w445 -> [w484]
                    tunnel: [w481] -> w444
                    tunnel: w443 -> [w471]
                    tunnel: w438 -> [w472]
                    tunnel: w439 -> [w473]
                    i -> [w483]
                    stop <- w482 continue-if-true
                    n168 = File/Directory Info(path=w473) -> (error out=w475:errorcluster)  [unwired: 1 in, 6 out]
                    n169 = File/Directory Info(path=w472) -> (error out=w476:errorcluster)  [unwired: 1 in, 6 out]
                    n170 = Unbundle By Name(w475) -> ("status"=w479:bool)
                    n171 = Unbundle By Name(w476) -> ("status"=w480:bool)
                    n172 = Empty String/Path?(string/path=w472) -> (empty?=w478:bool)
                    n173 = Empty String/Path?(string/path=w473) -> (empty?=w477:bool)
                    n174 = Compound Arithmetic op=AND(invert w479, invert w477, invert w480, invert w478) -> (w474:bool)
                    n175 = case shown="True" w474 {
                      tunnel: w484 -> [w485 w497]
                      tunnel: w472 -> [_ w496]
                      tunnel: w473 -> [_ w495]
                      tunnel: w483 -> [_ w493]
                      tunnel: [_ w490] -> w482
                      tunnel: w471 -> [_ w489]
                      tunnel: [w485 w486] -> w481
                      frame False {
                      }
                      frame True {
                        n176 = Build Array(w495) -> (w488:path[])
                        n177 = Build Array(w496) -> (w487:path[])
                        n178 = call <resource>:"Scripting_ReplaceVisAndControls.vi"("ViRef"=w489, "OldVIsAndControls"=w488, "NewVIsAndControls"=w487, "error in (no error)"=w497) -> ("error out"=w486:errorcluster)  [unwired: 14 in, 1 out]
                        n179 = Unbundle By Name(w486) -> ("status"=w494:bool)  [unwired: 1 out]
                        n180 = Less Or Equal?(x=w493, y=3) -> (x <= y?=w491:bool)
                        n181 = And(x=w491, y=w494) -> (x .and. y?=w490:bool)
                      }
                    }
                  }
                }
              }
            }
            n182 = Unbundle By Name(w387) -> ("TempClass"=w386:refnum<vi>)
            n183 = stacked-sequence {
              tunnel: w386 -> [w403]
              tunnel: w385 -> [_]
              frame #0 {
                n184 = Close Reference(reference=w403) -> ()  [unwired: 1 in, 1 out]
              }
            }
          }
          frame "AnyProtectedAttributesToUpdate?" {
            n185 = Unbundle By Name(w499) -> ("BaseClassFolder"=w517:path)
            n186 = Unbundle By Name(w499) -> ("VIs"=w522:refnum<vi>[])
            n187 = call <vilib>:"Recursive File List.vi"("Folder Path"=w517) -> ("All Files in Dir"=w506:path[])  [unwired: 6 in, 4 out]
            n188 = for {
              tunnel: w522 -> [w550] mode=indexing
              tunnel: [w549] -> w503 mode=indexing
              tunnel: [w547] -> w519 mode=indexing
              n189 = property class="VI"(reference=w550) -> ("Path"=w549:path)  [unwired: 1 in, 2 out]
              n190 = Strip Path(path=w549) -> (name=w548:string)  [unwired: 1 out]
              n191 = To Lower Case(string=w548) -> (all lower case string=w547:string)
            }
            n192 = for {
              tunnel: w506 -> [w535] mode=indexing
              tunnel: [w534] -> w512 mode=indexing
              n193 = Strip Path(path=w535) -> (name=w536:string)  [unwired: 1 out]
              n194 = To Lower Case(string=w536) -> (all lower case string=w534:string)
            }
            n195 = To Lower Case(string="ObjectAttributes.ctl") -> (all lower case string=w516:string)
            n196 = Unbundle By Name(w499) -> ("App"=w498:refnum<vi>)
            n197 = To Lower Case(string="ClassAttributes.ctl") -> (all lower case string=w511:string)
            n198 = Search 1D Array(1D array=w512, element=w516) -> (index of element=w507:i32)  [unwired: 1 in]
            n199 = Search 1D Array(1D array=w512, element=w511) -> (index of element=w505:i32)  [unwired: 1 in]
            n200 = Search 1D Array(1D array=w519, element=w516) -> (index of element=w508:i32)  [unwired: 1 in]
            n201 = Search 1D Array(1D array=w519, element=w511) -> (index of element=w502:i32)  [unwired: 1 in]
            n202 = Greater Or Equal To 0?(x=w505) -> (x >= 0?=w510:bool)
            n203 = Greater Or Equal To 0?(x=w507) -> (x >= 0?=w514:bool)
            n204 = Greater Or Equal To 0?(x=w508) -> (x >= 0?=w515:bool)
            n205 = Greater Or Equal To 0?(x=w502) -> (x >= 0?=w509:bool)
            n206 = And(x=w514, y=w515) -> (x .and. y?=w513:bool)
            n207 = And(x=w510, y=w509) -> (x .and. y?=w504:bool)
            n208 = case shown="True" w513 {
              tunnel: w520 -> [w545 w546]
              tunnel: w503 -> [w544 _]
              tunnel: w506 -> [w542 _]
              tunnel: w508 -> [w540 _]
              tunnel: w507 -> [w539 _]
              tunnel: [w538 w546] -> w501
              tunnel: w498 -> [w537 _]
              frame True {
                n209 = Index Array(array=w544, index=w540) -> (element=w543:path)
                n210 = Index Array(array=w542, index=w539) -> (element=w541:path)
                n211 = call <resource>:"Scripting_UpdateProtectedClassData.vi"("AppRef"=w537, "error in (no error)"=w545, "NewBaseAttribute"=w541, "BaseAttribute"=w543) -> ("error out"=w538:errorcluster)  [unwired: 6 in, 1 out]
              }
              frame False {
              }
            }
            n212 = case shown="True" w504 {
              tunnel: w503 -> [w532 _]
              tunnel: w506 -> [w530 _]
              tunnel: w502 -> [w528 _]
              tunnel: w505 -> [w527 _]
              tunnel: w501 -> [w526 w533]
              tunnel: [w525 w533] -> w500
              tunnel: w498 -> [w524 _]
              frame True {
                n213 = Index Array(array=w532, index=w528) -> (element=w531:path)
                n214 = Index Array(array=w530, index=w527) -> (element=w529:path)
                n215 = call <resource>:"Scripting_UpdateProtectedClassData.vi"("AppRef"=w524, "error in (no error)"=w526, "NewBaseAttribute"=w529, "BaseAttribute"=w531) -> ("error out"=w525:errorcluster)  [unwired: 6 in, 1 out]
              }
              frame False {
              }
            }
          }
          frame "AddFolders" {
            n216 = Unbundle By Name(w560) -> ("ClassRefnum"=w561:refnum<vi>)
            n217 = Unbundle By Name(w560) -> ("TemplateName"=w559:string)
            n218 = call <resource>:"UpdateClassApperance.vi"("ClassRefIn"=w561, "error in (no error)"=w562) -> ("error out"=w554:errorcluster)  [unwired: 16 in, 1 out]
            n219 = call <resource>:"GOOP400_ConfigurationMemory.vi"("error in (no error)"=w554, "Action"=enum16{"Read", "Load", "Save"}."Read") -> ("OptionsOut"=w552:T12, "error out"=w553:errorcluster)  [unwired: 16 in]
            n220 = Unbundle By Name(w552) -> ("FlatFolderStructure"=w551:bool)
            n221 = Match Pattern(string=w559, regular expression="Interface") -> (offset past match=w557:i32)  [unwired: 1 in, 3 out]
            n222 = Greater Or Equal To 0?(x=w557) -> (x >= 0?=w556:bool)
            n223 = case shown="False" w556 {
              tunnel: [w570 w580] -> w564
              tunnel: w553 -> [w568 w580]
              tunnel: w561 -> [w567 _]
              tunnel: w551 -> [w566 _]
              frame False {
                (unwired) TRUE ("CreateThePfysicalFolderIfPossible(False)")
                n224 = Not(x=w566) -> (.not. x?=w565:bool)
                n225 = call <resource>:"GDSProject_CreateFolder.vi"("Project Item To Create Folder Below(Use MyComputer if not wired)"=w567, "FolderName"="private", "error in (no error)"=w568, "CreateThePhysicalFolderIfPossible(False)"=w565) -> ("ItemOut"=w573:refnum<vi>, "FolderCreated"=w569:bool, "error out"=w571:errorcluster)  [unwired: 12 in, 1 out]
                n226 = case shown="True" w569 {
                  tunnel: w573 -> [_ w575]
                  tunnel: w571 -> [w574 w578]
                  tunnel: [w574 w576] -> w570
                  tunnel: w567 -> [_ w577]
                  frame False {
                  }
                  frame True {
                    n227 = invoke class="LVClassLibrary" method="Set Source Scope"(reference=w577, error in=w578, "SourceRef"=w575, "Scope"=T7."private" ("scope")) -> (error out=w576:errorcluster)  [unwired: 1 in, 4 out]
                    n228 = Close Reference(reference=w575, error in (no error)=w576) -> ()  [unwired: 1 out]
                  }
                }
              }
              frame True {
              }
            }
          }
          frame "CloseRefs", "Error", Default {
            n229 = case shown="\"CloseRefs\"" w599 {
              tunnel: w600 -> [w622 w626]
              tunnel: w583 -> [w621 w625]
              tunnel: [w622 w624] -> w584
              frame "False", Default {
                n230 = Unbundle By Name(w621) -> ("VIs"=w620:refnum<vi>[])
                n231 = Close Reference(reference=w620) -> ()  [unwired: 1 in, 1 out]
              }
              frame "CloseRefs" {
                n232 = Unbundle By Name(w625) -> ("ViLocked"=w623:bool[], "VIs"=w627:refnum<vi>[])
                n233 = for {
                  tunnel: w627 -> [w632] mode=indexing
                  shift-right: [w628] -> w624
                  shift-left: w626 -> [w633]
                  tunnel: w623 -> [w629] mode=indexing
                  n234 = case shown="True" w629 {
                    tunnel: w633 -> [w637 w643]
                    tunnel: w632 -> [w638 w642]
                    tunnel: [w637 w641] -> w631
                    tunnel: [w638 w640] -> w630
                    frame False {
                    }
                    frame True {
                      n235 = invoke class="VI" method="Lock State.Set"(reference=w642, error in=w643, "lockState"=T8."Locked (No Password)" ("Lock State")) -> (reference out=w640:refnum<vi>, error out=w641:errorcluster)  [unwired: 4 in, 5 out]
                    }
                  }
                  n236 = call <resource>:"Scripting_SaveVi.vi"("ForceResaving(False)"=TRUE, "error in (no error)"=w631, "VIRefToSaveIn"=w630) -> ("error out"=w636:errorcluster, "VIRefToSaveOut"=w635:refnum<vi>)  [unwired: 7 in]
                  n237 = Close Reference(reference=w635, error in (no error)=w636) -> (error out=w628:errorcluster)
                }
              }
            }
            n238 = Unbundle By Name(w583) -> ("TempClass"=w582:refnum<vi>)
            n239 = stacked-sequence {
              tunnel: w584 -> [w602]
              tunnel: [w602] -> w581
              tunnel: w582 -> [w603]
              frame #0 {
                n240 = Close Reference(reference=w603) -> ()  [unwired: 1 in, 1 out]
              }
            }
            n241 = Unbundle By Name(w583) -> ("DeleteFiles"=w594:path[], "App"=w586:refnum<vi>, "ProjectRefnum"=w597:refnum<vi>, "ClassRefnum"=w593:refnum<vi>)
            n242 = call <resource>:"GDSLvClass_SaveEverythingInClass.vi"("ClassRefIn"=w593, "error in"=w581) -> ("ClassRefOut"=w588:refnum<vi>, "error out"=w590:errorcluster)  [unwired: 16 in]
            n243 = case shown="True" w591 {
              tunnel: [w606 w607] -> w598
              tunnel: w590 -> [w605 w607]
              tunnel: w588 -> [w604 _]
              frame False {
                n244 = Close Reference(reference=w604, error in (no error)=w605) -> (error out=w606:errorcluster)
              }
              frame True {
              }
            }
            n245 = Close Reference(reference=w597, error in (no error)=w598) -> (error out=w587:errorcluster)
            n246 = Close Reference(reference=w586, error in (no error)=w587) -> (error out=w585:errorcluster)
            n247 = for {
              shift-right: [w618] -> w589
              shift-left: w585 -> [w619]
              tunnel: w594 -> [w617] mode=indexing
              tunnel: [w616] -> w592 mode=indexing
              n248 = Delete(path (use dialog)=w617, error in=w619) -> (error out=w618:errorcluster)  [unwired: 3 in, 2 out]
              n249 = Strip Path(path=w617) -> (stripped path=w616:path)  [unwired: 1 out]
            }
            n250 = for {
              tunnel: w592 -> [w612] mode=indexing
              n251 = List Folder(path=w612) -> (path out=w608:path, filenames=w611:string[], error out=w609:errorcluster)  [unwired: 3 in, 1 out]
              n252 = Empty Array?(array=w611) -> (empty?=w610:bool)
              n253 = case shown="True" w610 {
                tunnel: w609 -> [_ w615]
                tunnel: w608 -> [_ w614]
                tunnel: [_ w613] -> _
                frame False {
                }
                frame True {
                  n254 = Delete(path (use dialog)=w614, error in=w615) -> (error out=w613:errorcluster)  [unwired: 3 in, 2 out]
                }
              }
            }
            n255 = call <resource>:"GDSError_LogErrorInformation.vi"("State"=w595, "LocalVariableData"=w583, "error in (no error)"=w589) -> ("error out"=w596:errorcluster)  [unwired: 16 in]
          }
        }
        n256 = Equal?(x=w34, y="Exit") -> (x = y?=w38:bool)
        n257 = Select(t="Error", s=w33, f=w34) -> (s? t:f=w37:string)
      }
      n258 = Unbundle By Name(w14) -> ("ClassRefnum"=w17:refnum<vi>, "TemplateVersion"=w16:string)
    }
    frame Error {
    }
  }
  "error out" <- w11
  "LVClassLibraryRefnum" <- w4
  "TemplateVersionUsed" <- w3
  "ClassWriterGOOP400.lvclass" <- "ClassWriterGOOP400.lvclass"
